vi "VISA Name to Base Value.vi"(1 "String":string) -> (0 "String 2":string)   [LabVIEW 2020]
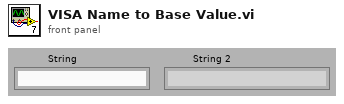
[diagram p1: front panel]
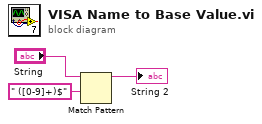
[diagram p0: block diagram]
diagram:
  n1 = Match Pattern(string="String", regular expression=" ([0-9]+)$") -> (before substring=→"String 2":string)  [unwired: 1 in, 3 out]
